vi "LCA Move To Pos.vi"(8 "error in (no error)":errorcluster caption="Fehler (Eingang, kein Fehler)", 9 "Velocity":dbl, 10 "Position":dbl, 11 "Axis Handle":i64) -> (0 "error out":errorcluster caption="Fehler (Ausgang)")   [LabVIEW 2021, in "labbCAN_MotionControl_API.lvlib"]
doc: "LCA_Func long __stdcall LCA_MoveToPos(dev_hdl hAxis,\n double fPosition,\n double fVelocity,\n unsigned long PrivData);"
uses:
  labbCAN_MotionControl_API.lvlib
  labbCAN_MotionControl_API.dll
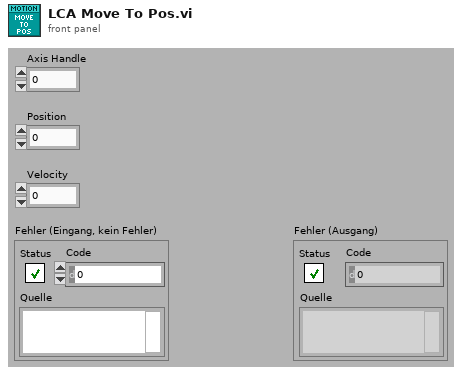
[diagram p1: front panel]
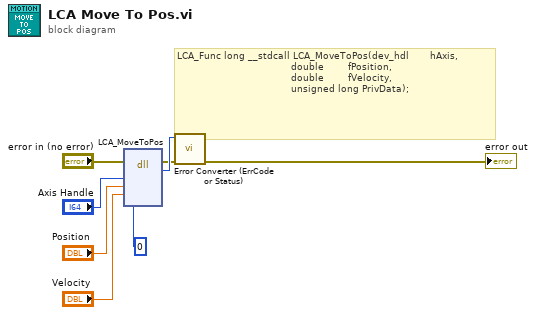
[diagram p0: block diagram]
diagram:
  # "LCA_Func long __stdcall LCA_MoveToPos(dev_hdl       hAxis,\n                                      double        fPosition,\n                                      double        fVelocity,\n                                      unsigned long PrivData);"
  n1 = dll-call lib="C:/Users/olaja/AppData/Local/CETONI_SDK/labbCAN_MotionControl_API.*" fn="LCA_MoveToPos"(error in="error in (no error)", "hAxis"="Axis Handle", "fPosition"="Position", "fVelocity"="Velocity", "PrivData"=u32 0) -> (error out=w3:errorcluster, "Rückgabetyp"=w8:i32)  [unwired: 6 in, 1 out]
  n2 = call "Error Converter (ErrCode or Status).vi"("error in (no error)"=w3, "error code"=w8) -> ("error out"=→"error out":errorcluster)  [unwired: 9 in]
